vi "Get Clock Time (seconds).vi"(8 "error in (no error)":errorcluster, 11 "clock id (monotonic)":T1=enum."Monotonic") -> (0 "error out":errorcluster, 3 "clock time (seconds)":dbl format="%.6g")   [LabVIEW 2013, in "Linux RT Utilities.lvlib"]
uses:
  Linux RT Utilities.lvlib
  Controls/Public/C Enums/clockid_t.ctl
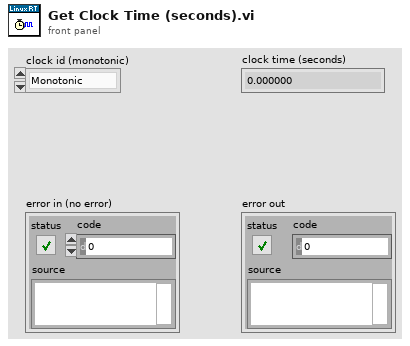
[diagram p1: front panel]
types:
  T1 = typedef "Linux RT Utilities.lvlib/clockid_t.ctl" = enum16{"Realtime", "Monotonic"}
  T2 = typedef "Linux RT Utilities.lvlib/timespec_64.ctl" = cluster{"sec":u64, "nsec":u64}
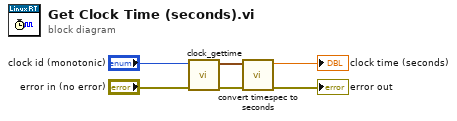
[diagram p0: block diagram]
diagram:
  n1 = call "clock_gettime.vi"("error in (no error)"="error in (no error)", "clock id (monotonic)"="clock id (monotonic)") -> ("error out"=→"error out":errorcluster, "timespec"=w3:T2)  [unwired: 8 in]
  n2 = call "convert timespec to seconds.vi"("timespec"=w3) -> ("seconds"=→"clock time (seconds)":dbl)  [unwired: 10 in]
